vi "Create_Trajectory_Config_Parse_V1_V2_V3.vi"(8 "error in (no error)":errorcluster, 10 "Units Selector":T4, 11 "XML Elements":string) -> (0 "error out":errorcluster, 3 "TrajCreateConfig":T1 {"WayPoints"."WEIGHT" format="%13.3f"; "WayPoints"."ANGLE" format="%13.3f"; "WayPoints"."Y" format="%13.3f"; "WayPoints"."X" format="%13.3f"; "TRAJECTORY_CONFIG"."End Velocity" format="%20.4f"; "TRAJECTORY_CONFIG"."StartVelocity" format="%20.4f"; "TRAJECTORY_CONFIG"."Max Acceleration" format="%20.4f"; "TRAJECTORY_CONFIG"."MaxVelocity" format="%20.4f"})   [LabVIEW 2019]
uses:
  CreateTrajectoryENUM/TrajCreateUnitsENUM.ctl
  CreateTrajectoryTypeDef/TrajCreateConfig__V_Internal.ctl
  <vilib>/Rock Robotics/WPI/ThirdParty/JAS_Junk/TrajLib/TypeDef/DISPLAY_WEIGHTED_WAYPOINT.ctl
  <vilib>/Rock Robotics/WPI/ThirdParty/JAS_Junk/TrajLib/TypeDef/TRAJ_CONFIG.ctl
  CreateTrajectoryTypeDef/TrajCreateConfig_V5.ctl
  CreateTrajectoryTypeDef/TrajCreateTrajConfig_V4.ctl
  <vilib>/Rock Robotics/WPI/ThirdParty/JAS_Junk/TrajLib/TypeDef/TRAJ_CONSTRAINT_DIIF_DRIVE_KINEMATICS.ctl
  <vilib>/Rock Robotics/WPI/ThirdParty/JAS_Junk/TrajLib/TypeDef/DIFF_DRIVE_KINEMATICS.ctl
  <vilib>/Rock Robotics/WPI/ThirdParty/JAS_Junk/TrajLib/TypeDef/TRAJ_CONSTRAINT_CENTRIPETAL_ACCEL.ctl
  <vilib>/Rock Robotics/WPI/ThirdParty/JAS_Junk/TrajLib/TypeDef/TRAJ_CONSTRAINT_SWERVE_DRIVE_KINEMATICS.ctl
  <vilib>/Rock Robotics/WPI/ThirdParty/JAS_Junk/TrajLib/TypeDef/SWERVE_DRIVE_KINEMATICS.ctl
  <vilib>/Analysis/Matrix/Datatypes/RealMatrix.ctl
  <vilib>/Rock Robotics/WPI/ThirdParty/JAS_Junk/TrajLib/TypeDef/TRANSLATION2D.ctl
  <vilib>/Rock Robotics/WPI/ThirdParty/JAS_Junk/TrajLib/TypeDef/SWERVE_DRIVE_MODULE_STATE.ctl
  <vilib>/Rock Robotics/WPI/ThirdParty/JAS_Junk/TrajLib/TypeDef/ROTATION2D.ctl
  <vilib>/Rock Robotics/WPI/ThirdParty/JAS_Junk/TrajLib/TypeDef/TRAJ_CONSTRAINT_DIIF_DRIVE_VOLTAGE.ctl
  <vilib>/Rock Robotics/WPI/ThirdParty/JAS_Junk/TrajLib/TypeDef/SIMPLE_MOTOR_FF.ctl
  <vilib>/Rock Robotics/WPI/ThirdParty/JAS_Junk/TrajLib/TypeDef/TRAJ_CONSTRAINT_MECA_DRIVE_KINEMATICS.ctl
  <vilib>/Rock Robotics/WPI/ThirdParty/JAS_Junk/TrajLib/TypeDef/MECA_DRIVE_KINEMATICS.ctl
  CreateTrajectoryTypeDef/TrajCreateConfig_V4.ctl
  CreateTrajectoryTypeDef/TrajCreateConfig_V3.ctl
  CreateTrajectoryTypeDef/TrajCreateConfig_V2.ctl
  <vilib>/Rock Robotics/WPI/ThirdParty/JAS_Junk/TrajLib/TypeDef/DISPLAY_WAYPOINT.ctl
  CreateTrajectoryTypeDef/TrajCreateConfig_V1.ctl
  <vilib>/Rock Robotics/WPI/ThirdParty/JAS_Junk/TrajLib/Trajectory_Library.lvlib
  <vilib>/Analysis/Matrix/NI_Matrix.lvlib
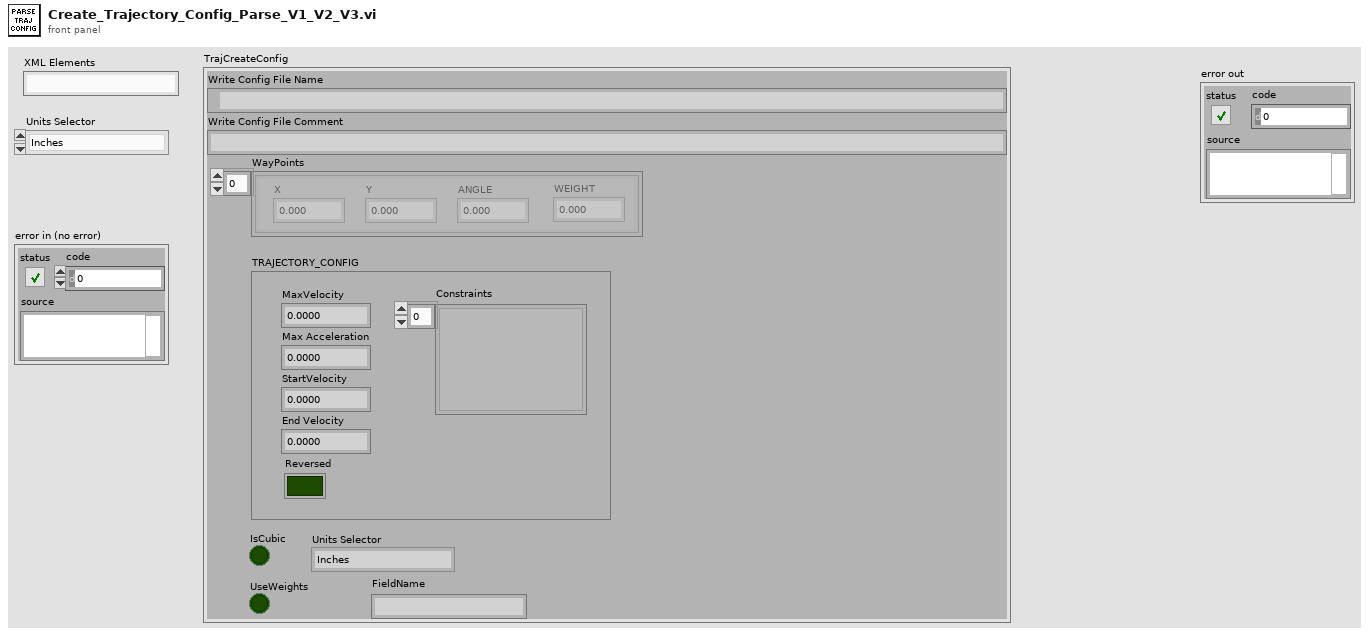
[diagram p1: front panel]
types:
  T1 = typedef "TrajCreateConfig__V_Internal.ctl" = cluster{"Write Config File Name":path, "Write Config File Comment":string, "WayPoints":T2[], "TRAJECTORY_CONFIG":T3, "IsCubic":bool, "Units Selector":T4, "UseWeights":bool, "FieldName":string}
  T2 = typedef "Trajectory_Library.lvlib/DISPLAY_WEIGHTED_WAYPOINT.ctl" = cluster{"X":dbl, "Y":dbl, "ANGLE":dbl, "WEIGHT":dbl}
  T3 = typedef "Trajectory_Library.lvlib/TRAJ_CONFIG.ctl" = cluster{"MaxVelocity":dbl, "Max Acceleration":dbl, "StartVelocity":dbl, "End Velocity":dbl, "Reversed":bool, "Constraints":variant[]}
  T4 = typedef "TrajCreateUnitsENUM.ctl" = enum16{"Inches", "Feet", "Centimeters", "Meters"}
  T5 = typedef "TrajCreateConfig_V5.ctl" = cluster{"Write Config File Name":path, "Write Config File Comment":string, "WayPoints":T2[], "TRAJECTORY_CONFIG_V4":T6, "IsCubic":bool, "Units Selector":T4, "UseWeights":bool, "FieldName":string, "Rect Region Exists":bool, "RectRegionBotLeft":T13, "RectRegionTopRight":T13, "Rect Region Max Speed":dbl}
  T6 = typedef "TrajCreateTrajConfig_V4.ctl" = cluster{"MaxVelocity":dbl, "Max Acceleration":dbl, "StartVelocity":dbl, "End Velocity":dbl, "Reversed":bool, "DiffDrKineConstntDefined":bool, "CentAcellConstntDefined":bool, "DiffDrVoltConstntDefined":bool, "DIFF_DRIVE_KINE_CONSTRAINT":T7, "CENTRIPETAL_ACCEL_CONSTRAINT":T9, "SwerveDrKineConstntDefined":bool, "SWERVE_DRIVE_KINE_CONSTRAINT":T10, "DIFF_DRIVE_VOLTAGE_CONSTRAINT":T16, "MECANUM_DRIVE_KINE_CONSTRAINT":T18, "MecanumDrKineConstntDefined":bool}
  T7 = typedef "Trajectory_Library.lvlib/TRAJ_CONSTRAINT_DIIF_DRIVE_KINEMATICS.ctl" = cluster{"Max Speed (M/S)":dbl, "DIFF_DRIVE_KINEMATICS":T8, "Max Accel (M/S2)":dbl}
  T8 = typedef "Trajectory_Library.lvlib/DIFF_DRIVE_KINEMATICS.ctl" = cluster{"TrackWidth_Meters":dbl}
  T9 = typedef "Trajectory_Library.lvlib/TRAJ_CONSTRAINT_CENTRIPETAL_ACCEL.ctl" = cluster{"Max Cent Accel":dbl}
  T10 = typedef "Trajectory_Library.lvlib/TRAJ_CONSTRAINT_SWERVE_DRIVE_KINEMATICS.ctl" = cluster{"Max Speed (M/S)":dbl, "SwerveKinematics":T11}
  T11 = typedef "Trajectory_Library.lvlib/SWERVE_DRIVE_KINEMATICS.ctl" = cluster{"NumModules":i32, "InverseKinematics":T12, "ForwardKinematics":T12, "Modules":T13[], "PrevCoR":T13, "SavedModuleStates":T14[]}
  T12 = typedef "NI_Matrix.lvlib/RealMatrix.ctl" = dbl[][]
  T13 = typedef "Trajectory_Library.lvlib/TRANSLATION2D.ctl" = cluster{"X":dbl, "Y":dbl}
  T14 = typedef "Trajectory_Library.lvlib/SWERVE_DRIVE_MODULE_STATE.ctl" = cluster{"Speed":dbl, "Angle":T15}
  T15 = typedef "Trajectory_Library.lvlib/ROTATION2D.ctl" = cluster{"VALUE":dbl, "COS":dbl, "SIN":dbl}
  T16 = typedef "Trajectory_Library.lvlib/TRAJ_CONSTRAINT_DIIF_DRIVE_VOLTAGE.ctl" = cluster{"Max Voltage":dbl, "DIFF_DRIVE_KINEMATICS":T8, "SIMPLE_MOTOR_FF":T17}
  T17 = typedef "Trajectory_Library.lvlib/SIMPLE_MOTOR_FF.ctl" = cluster{"Ks":dbl, "Kv":dbl, "Ka":dbl, "KnInv":dbl}
  T18 = typedef "Trajectory_Library.lvlib/TRAJ_CONSTRAINT_MECA_DRIVE_KINEMATICS.ctl" = cluster{"Max Speed (M/S)":dbl, "MECA_DRIVE_KINEMATICS":T19}
  T19 = typedef "Trajectory_Library.lvlib/MECA_DRIVE_KINEMATICS.ctl" = cluster{"FrontLeft":T13, "FrontRight":T13, "RearLeft":T13, "RearRight":T13, "InverseKinematics":T12, "ForwardKinematics":T12, "PrevCoR":T13}
  T20 = typedef "TrajCreateConfig_V4.ctl" = cluster{"Write Config File Name":path, "Write Config File Comment":string, "WayPoints":T2[], "TRAJECTORY_CONFIG_V4":T6, "IsCubic":bool, "Units Selector":T4, "UseWeights":bool, "FieldName":string}
  T21 = typedef "TrajCreateConfig_V3.ctl" = cluster{"Write Config File Name":path, "Write Config File Comment":string, "WayPoints":T2[], "TRAJECTORY_CONFIG":cluster{"MaxVelocity":dbl, "Max Acceleration":dbl, "StartVelocity":dbl, "End Velocity":dbl, "Reversed":bool, "DiffDrKineConstntDefined":bool, "CentAcellConstntDefined":bool, "DiffDrVoltConstntDefined":bool, "DIFF_DRIVE_KINE_CONSTRAINT":cluster{"Max Speed (M/S)":dbl, "DIFF_DRIVE_KINEMATICS":T8}, "CENTRIPETAL_ACCEL_CONSTRAINT":T9, "SwerveDrKineConstntDefined":bool, "SWERVE_DRIVE_KINE_CONSTRAINT":T10, "DIFF_DRIVE_VOLTAGE_CONSTRAINT":T16, "MECANUM_DRIVE_KINE_CONSTRAINT":T18, "MecanumDrKineConstntDefined":bool}, "IsCubic":bool, "Units Selector":T4, "UseWeights":bool}
  T22 = typedef "TrajCreateConfig_V2.ctl" = cluster{"Write Config File Name":path, "Write Config File Comment":string, "WayPoints":T23[], "TRAJECTORY_CONFIG":cluster{"MaxVelocity":dbl, "Max Acceleration":dbl, "StartVelocity":dbl, "End Velocity":dbl, "Reversed":bool, "DiffDrKineConstntDefined":bool, "CentAcellConstntDefined":bool, "DiffDrVoltConstntDefined":bool, "DIFF_DRIVE_KINE_CONSTRAINT":cluster{"Max Speed (M/S)":dbl, "DIFF_DRIVE_KINEMATICS":T8}, "CENTRIPETAL_ACCEL_CONSTRAINT":T9, "SwerveDrKineConstntDefined":bool, "SWERVE_DRIVE_KINE_CONSTRAINT":T10, "DIFF_DRIVE_VOLTAGE_CONSTRAINT":T16, "MECANUM_DRIVE_KINE_CONSTRAINT":T18, "MecanumDrKineConstntDefined":bool}, "IsCubic":bool, "Units Selector":T4}
  T23 = typedef "Trajectory_Library.lvlib/DISPLAY_WAYPOINT.ctl" = cluster{"X":dbl, "Y":dbl, "ANGLE":dbl}
  T24 = typedef "TrajCreateConfig_V1.ctl" = cluster{"Write Config File Name":path, "Write Config File Comment":string, "WayPoints":T23[], "TRAJECTORY_CONFIG":cluster{"MaxVelocity":dbl, "Max Acceleration":dbl, "StartVelocity":dbl, "End Velocity":dbl, "Reversed":bool, "DiffDrKineConstntDefined":bool, "CentAcellConstntDefined":bool, "DiffDrVoltConstntDefined":bool, "DIFF_DRIVE_KINE_CONSTRAINT":cluster{"Max Speed (M/S)":dbl, "DIFF_DRIVE_KINEMATICS":T8}, "CENTRIPETAL_ACCEL_CONSTRAINT":T9, "SwerveDrKineConstntDefined":bool, "SWERVE_DRIVE_KINE_CONSTRAINT":T10, "DIFF_DRIVE_VOLTAGE_CONSTRAINT":T16, "MECANUM_DRIVE_KINE_CONSTRAINT":T18, "MecanumDrKineConstntDefined":bool}, "IsCubic":bool}
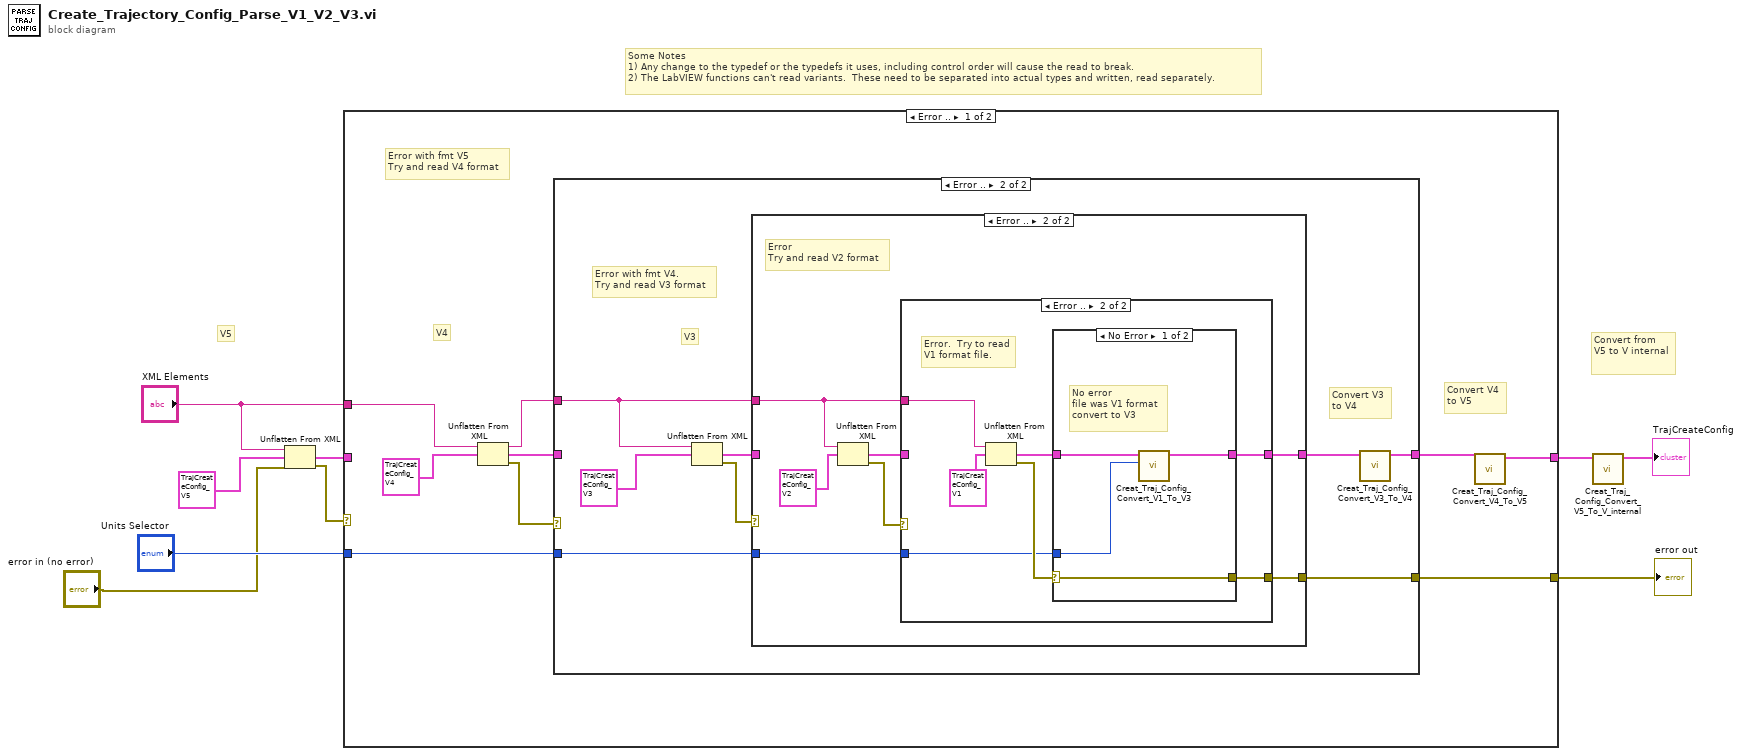
[diagram p0: block diagram]
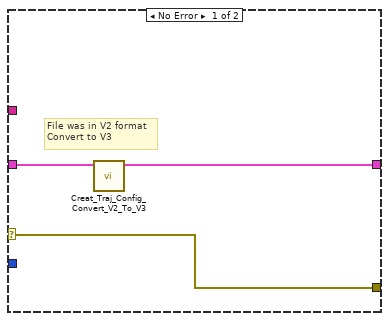
[diagram p4: hidden frame]
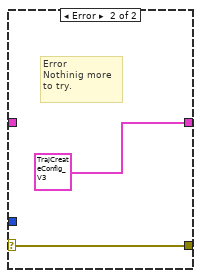
[diagram p5: hidden frame]
diagram:
  # "V5"
  # "Convert from\nV5 to V internal"
  # "Some Notes\n1) Any change to the typedef or the typedefs it uses, including control order will cause the read to break.\n2) The LabVIEW functions can't read variants.  These need to be separated into actual types and written, read separately."
  n1 = Unflatten From XML(xml string="XML Elements", type=T5 {"Write Config File Name"=path "", "Write Config File Comment"="", "WayPoints"=[], "TRAJECTORY_CONFIG_V4"={"MaxVelocity"=0.0, "Max Acceleration"=0.0, "StartVelocity"=0.0, "End Velocity"=0.0, "Reversed"=FALSE, "DiffDrKineConstntDefined"=FALSE, "CentAcellConstntDefined"=FALSE, "DiffDrVoltConstntDefined"=FALSE, "DIFF_DRIVE_KINE_CONSTRAINT"={"Max Speed (M/S)"=0.0, "DIFF_DRIVE_KINEMATICS"={"TrackWidth_Meters"=0.0}, "Max Accel (M/S2)"=99999.0}, "CENTRIPETAL_ACCEL_CONSTRAINT"={"Max Cent Accel"=0.0}, "SwerveDrKineConstntDefined"=FALSE, "SWERVE_DRIVE_KINE_CONSTRAINT"={"Max Speed (M/S)"=0.0, "SwerveKinematics"={"NumModules"=0, "InverseKinematics"=[], "ForwardKinematics"=[], "Modules"=[], "PrevCoR"={"X"=0.0, "Y"=0.0}, "SavedModuleStates"=[]}}, "DIFF_DRIVE_VOLTAGE_CONSTRAINT"={"Max Voltage"=0.0, "DIFF_DRIVE_KINEMATICS"={"TrackWidth_Meters"=0.0}, "SIMPLE_MOTOR_FF"={"Ks"=0.0, "Kv"=0.0, "Ka"=0.0, "KnInv"=0.0}}, "MECANUM_DRIVE_KINE_CONSTRAINT"={"Max Speed (M/S)"=0.0, "MECA_DRIVE_KINEMATICS"={"FrontLeft"={"X"=0.0, "Y"=0.0}, "FrontRight"={"X"=0.0, "Y"=0.0}, "RearLeft"={"X"=0.0, "Y"=0.0}, "RearRight"={"X"=0.0, "Y"=0.0}, "InverseKinematics"=[[0.0, 1.0, -1.0, 0.0], [0.0, 1.0, 1.0, 0.0], [0.0, 1.0, 1.0, 0.0], [0.0, 1.0, -1.0, 0.0]], "ForwardKinematics"=[[0.0, 1.0, -1.0, 0.0], [0.0, 1.0, 1.0, 0.0], [0.0, 1.0, 1.0, 0.0], [0.0, 1.0, -1.0, 0.0]], "PrevCoR"={"X"=0.0, "Y"=0.0}}}, "MecanumDrKineConstntDefined"=FALSE}, "IsCubic"=FALSE, "Units Selector"=enum."Inches", "UseWeights"=FALSE, "FieldName"="", "Rect Region Exists"=FALSE, "RectRegionBotLeft"={"X"=0.0, "Y"=0.0}, "RectRegionTopRight"={"X"=0.0, "Y"=0.0}, "Rect Region Max Speed"=0.0} ("TrajCreateConfigV5"), error in (no error)="error in (no error)") -> (value=w2:T5, error out=w6:errorcluster)
  n2 = case shown="Error .." w6 {
    selector: w6 -> [_ w53]
    tunnel: "Units Selector" -> [w17 _]
    tunnel: [w16 w53] -> w8
    tunnel: "XML Elements" -> [w13 _]
    tunnel: w2 -> [_ w54]
    tunnel: [w10 w54] -> w1
    frame Error {
      # "V4"
      # "Convert V4\nto V5"
      # "Error with fmt V5\nTry and read V4 format"
      n3 = Unflatten From XML(xml string=w13, type=T20 {"Write Config File Name"=path "", "Write Config File Comment"="", "WayPoints"=[], "TRAJECTORY_CONFIG_V4"={"MaxVelocity"=0.0, "Max Acceleration"=0.0, "StartVelocity"=0.0, "End Velocity"=0.0, "Reversed"=FALSE, "DiffDrKineConstntDefined"=FALSE, "CentAcellConstntDefined"=FALSE, "DiffDrVoltConstntDefined"=FALSE, "DIFF_DRIVE_KINE_CONSTRAINT"={"Max Speed (M/S)"=0.0, "DIFF_DRIVE_KINEMATICS"={"TrackWidth_Meters"=0.0}, "Max Accel (M/S2)"=99999.0}, "CENTRIPETAL_ACCEL_CONSTRAINT"={"Max Cent Accel"=0.0}, "SwerveDrKineConstntDefined"=FALSE, "SWERVE_DRIVE_KINE_CONSTRAINT"={"Max Speed (M/S)"=0.0, "SwerveKinematics"={"NumModules"=0, "InverseKinematics"=[], "ForwardKinematics"=[], "Modules"=[], "PrevCoR"={"X"=0.0, "Y"=0.0}, "SavedModuleStates"=[]}}, "DIFF_DRIVE_VOLTAGE_CONSTRAINT"={"Max Voltage"=0.0, "DIFF_DRIVE_KINEMATICS"={"TrackWidth_Meters"=0.0}, "SIMPLE_MOTOR_FF"={"Ks"=0.0, "Kv"=0.0, "Ka"=0.0, "KnInv"=0.0}}, "MECANUM_DRIVE_KINE_CONSTRAINT"={"Max Speed (M/S)"=0.0, "MECA_DRIVE_KINEMATICS"={"FrontLeft"={"X"=0.0, "Y"=0.0}, "FrontRight"={"X"=0.0, "Y"=0.0}, "RearLeft"={"X"=0.0, "Y"=0.0}, "RearRight"={"X"=0.0, "Y"=0.0}, "InverseKinematics"=[[0.0, 1.0, -1.0, 0.0], [0.0, 1.0, 1.0, 0.0], [0.0, 1.0, 1.0, 0.0], [0.0, 1.0, -1.0, 0.0]], "ForwardKinematics"=[[0.0, 1.0, -1.0, 0.0], [0.0, 1.0, 1.0, 0.0], [0.0, 1.0, 1.0, 0.0], [0.0, 1.0, -1.0, 0.0]], "PrevCoR"={"X"=0.0, "Y"=0.0}}}, "MecanumDrKineConstntDefined"=FALSE}, "IsCubic"=FALSE, "Units Selector"=enum."Inches", "UseWeights"=FALSE, "FieldName"=""} ("TrajCreateConfig")) -> (value=w12:T20, error out=w14:errorcluster)  [unwired: 1 in]
      n4 = case shown="Error .." w14 {
        selector: w14 -> [w18 _]
        tunnel: w17 -> [_ w27]
        tunnel: [w18 w26] -> w16
        tunnel: w13 -> [_ w22]
        tunnel: [w19 w20] -> w11
        tunnel: w12 -> [w19 _]
        frame No Error {
          # "No Error -- File was in V4 Format"
        }
        frame Error {
          # "Convert V3\nto V4"
          # "Error with fmt V4.\nTry and read V3 format"
          # "V3"
          n5 = Unflatten From XML(xml string=w22, type=T21 {"Write Config File Name"=path "", "Write Config File Comment"="", "WayPoints"=[], "TRAJECTORY_CONFIG"={"MaxVelocity"=0.0, "Max Acceleration"=0.0, "StartVelocity"=0.0, "End Velocity"=0.0, "Reversed"=FALSE, "DiffDrKineConstntDefined"=FALSE, "CentAcellConstntDefined"=FALSE, "DiffDrVoltConstntDefined"=FALSE, "DIFF_DRIVE_KINE_CONSTRAINT"={"Max Speed (M/S)"=0.0, "DIFF_DRIVE_KINEMATICS"={"TrackWidth_Meters"=0.0}}, "CENTRIPETAL_ACCEL_CONSTRAINT"={"Max Cent Accel"=0.0}, "SwerveDrKineConstntDefined"=FALSE, "SWERVE_DRIVE_KINE_CONSTRAINT"={"Max Speed (M/S)"=0.0, "SwerveKinematics"={"NumModules"=0, "InverseKinematics"=[], "ForwardKinematics"=[], "Modules"=[], "PrevCoR"={"X"=0.0, "Y"=0.0}, "SavedModuleStates"=[]}}, "DIFF_DRIVE_VOLTAGE_CONSTRAINT"={"Max Voltage"=0.0, "DIFF_DRIVE_KINEMATICS"={"TrackWidth_Meters"=0.0}, "SIMPLE_MOTOR_FF"={"Ks"=0.0, "Kv"=0.0, "Ka"=0.0, "KnInv"=0.0}}, "MECANUM_DRIVE_KINE_CONSTRAINT"={"Max Speed (M/S)"=0.0, "MECA_DRIVE_KINEMATICS"={"FrontLeft"={"X"=0.0, "Y"=0.0}, "FrontRight"={"X"=0.0, "Y"=0.0}, "RearLeft"={"X"=0.0, "Y"=0.0}, "RearRight"={"X"=0.0, "Y"=0.0}, "InverseKinematics"=[], "ForwardKinematics"=[], "PrevCoR"={"X"=0.0, "Y"=0.0}}}, "MecanumDrKineConstntDefined"=FALSE}, "IsCubic"=FALSE, "Units Selector"=enum."Inches", "UseWeights"=FALSE} ("TrajCreateConfig")) -> (value=w24:T21, error out=w23:errorcluster)  [unwired: 1 in]
          n6 = case shown="Error .." w23 {
            selector: w23 -> [w29 _]
            tunnel: [w29 w32] -> w26
            tunnel: w27 -> [_ w34]
            tunnel: w24 -> [w28 _]
            tunnel: [w28 w31] -> w21
            tunnel: w22 -> [_ w30]
            frame No Error {
              # "No Error.  File was V3\nformat."
            }
            frame Error {
              # "Error\nTry and read V2 format"
              n7 = Unflatten From XML(xml string=w30, type=T22 {"Write Config File Name"=path "", "Write Config File Comment"="", "WayPoints"=[], "TRAJECTORY_CONFIG"={"MaxVelocity"=0.0, "Max Acceleration"=0.0, "StartVelocity"=0.0, "End Velocity"=0.0, "Reversed"=FALSE, "DiffDrKineConstntDefined"=FALSE, "CentAcellConstntDefined"=FALSE, "DiffDrVoltConstntDefined"=FALSE, "DIFF_DRIVE_KINE_CONSTRAINT"={"Max Speed (M/S)"=0.0, "DIFF_DRIVE_KINEMATICS"={"TrackWidth_Meters"=0.0}}, "CENTRIPETAL_ACCEL_CONSTRAINT"={"Max Cent Accel"=0.0}, "SwerveDrKineConstntDefined"=FALSE, "SWERVE_DRIVE_KINE_CONSTRAINT"={"Max Speed (M/S)"=0.0, "SwerveKinematics"={"NumModules"=0, "InverseKinematics"=[], "ForwardKinematics"=[], "Modules"=[], "PrevCoR"={"X"=0.0, "Y"=0.0}, "SavedModuleStates"=[]}}, "DIFF_DRIVE_VOLTAGE_CONSTRAINT"={"Max Voltage"=0.0, "DIFF_DRIVE_KINEMATICS"={"TrackWidth_Meters"=0.0}, "SIMPLE_MOTOR_FF"={"Ks"=0.0, "Kv"=0.0, "Ka"=0.0, "KnInv"=0.0}}, "MECANUM_DRIVE_KINE_CONSTRAINT"={"Max Speed (M/S)"=0.0, "MECA_DRIVE_KINEMATICS"={"FrontLeft"={"X"=0.0, "Y"=0.0}, "FrontRight"={"X"=0.0, "Y"=0.0}, "RearLeft"={"X"=0.0, "Y"=0.0}, "RearRight"={"X"=0.0, "Y"=0.0}, "InverseKinematics"=[], "ForwardKinematics"=[], "PrevCoR"={"X"=0.0, "Y"=0.0}}}, "MecanumDrKineConstntDefined"=FALSE}, "IsCubic"=FALSE, "Units Selector"=enum."Inches"} ("TrajCreateConfig")) -> (value=w35:T22, error out=w33:errorcluster)  [unwired: 1 in]
              n8 = case shown="Error .." w33 {
                selector: w33 -> [w38 _]
                tunnel: w35 -> [w39 _]
                tunnel: w34 -> [_ w41]
                tunnel: [w38 w43] -> w32
                tunnel: [w37 w42] -> w31
                tunnel: w30 -> [_ w45]
                frame No Error {
                  # "File was in V2 format\nConvert to V3"
                  n9 = call "Creat_Traj_Config_Convert_V2_To_V3.vi"("TrajCreateConfig in"=w39) -> ("TrajCreateConfig out"=w37:T21)  [unwired: 10 in]
                }
                frame Error {
                  # "Error.  Try to read\nV1 format file."
                  n10 = Unflatten From XML(xml string=w45, type=T24 {"Write Config File Name"=path "", "Write Config File Comment"="", "WayPoints"=[], "TRAJECTORY_CONFIG"={"MaxVelocity"=0.0, "Max Acceleration"=0.0, "StartVelocity"=0.0, "End Velocity"=0.0, "Reversed"=FALSE, "DiffDrKineConstntDefined"=FALSE, "CentAcellConstntDefined"=FALSE, "DiffDrVoltConstntDefined"=FALSE, "DIFF_DRIVE_KINE_CONSTRAINT"={"Max Speed (M/S)"=0.0, "DIFF_DRIVE_KINEMATICS"={"TrackWidth_Meters"=0.0}}, "CENTRIPETAL_ACCEL_CONSTRAINT"={"Max Cent Accel"=0.0}, "SwerveDrKineConstntDefined"=FALSE, "SWERVE_DRIVE_KINE_CONSTRAINT"={"Max Speed (M/S)"=0.0, "SwerveKinematics"={"NumModules"=0, "InverseKinematics"=[], "ForwardKinematics"=[], "Modules"=[], "PrevCoR"={"X"=0.0, "Y"=0.0}, "SavedModuleStates"=[]}}, "DIFF_DRIVE_VOLTAGE_CONSTRAINT"={"Max Voltage"=0.0, "DIFF_DRIVE_KINEMATICS"={"TrackWidth_Meters"=0.0}, "SIMPLE_MOTOR_FF"={"Ks"=0.0, "Kv"=0.0, "Ka"=0.0, "KnInv"=0.0}}, "MECANUM_DRIVE_KINE_CONSTRAINT"={"Max Speed (M/S)"=0.0, "MECA_DRIVE_KINEMATICS"={"FrontLeft"={"X"=0.0, "Y"=0.0}, "FrontRight"={"X"=0.0, "Y"=0.0}, "RearLeft"={"X"=0.0, "Y"=0.0}, "RearRight"={"X"=0.0, "Y"=0.0}, "InverseKinematics"=[], "ForwardKinematics"=[], "PrevCoR"={"X"=0.0, "Y"=0.0}}}, "MecanumDrKineConstntDefined"=FALSE}, "IsCubic"=FALSE} ("TrajCreateConfig")) -> (value=w40:T24, error out=w44:errorcluster)  [unwired: 1 in]
                  n11 = case shown="No Error" w44 {
                    selector: w44 -> [w50 w52]
                    tunnel: [w50 w52] -> w43
                    tunnel: [w49 T21 {"Write Config File Name"=path "", "Write Config File Comment"="", "WayPoints"=[], "TRAJECTORY_CONFIG"={"MaxVelocity"=0.0, "Max Acceleration"=0.0, "StartVelocity"=0.0, "End Velocity"=0.0, "Reversed"=FALSE, "DiffDrKineConstntDefined"=FALSE, "CentAcellConstntDefined"=FALSE, "DiffDrVoltConstntDefined"=FALSE, "DIFF_DRIVE_KINE_CONSTRAINT"={"Max Speed (M/S)"=0.0, "DIFF_DRIVE_KINEMATICS"={"TrackWidth_Meters"=0.0}}, "CENTRIPETAL_ACCEL_CONSTRAINT"={"Max Cent Accel"=0.0}, "SwerveDrKineConstntDefined"=FALSE, "SWERVE_DRIVE_KINE_CONSTRAINT"={"Max Speed (M/S)"=0.0, "SwerveKinematics"={"NumModules"=0, "InverseKinematics"=[], "ForwardKinematics"=[], "Modules"=[], "PrevCoR"={"X"=0.0, "Y"=0.0}, "SavedModuleStates"=[]}}, "DIFF_DRIVE_VOLTAGE_CONSTRAINT"={"Max Voltage"=0.0, "DIFF_DRIVE_KINEMATICS"={"TrackWidth_Meters"=0.0}, "SIMPLE_MOTOR_FF"={"Ks"=0.0, "Kv"=0.0, "Ka"=0.0, "KnInv"=0.0}}, "MECANUM_DRIVE_KINE_CONSTRAINT"={"Max Speed (M/S)"=0.0, "MECA_DRIVE_KINEMATICS"={"FrontLeft"={"X"=0.0, "Y"=0.0}, "FrontRight"={"X"=0.0, "Y"=0.0}, "RearLeft"={"X"=0.0, "Y"=0.0}, "RearRight"={"X"=0.0, "Y"=0.0}, "InverseKinematics"=[], "ForwardKinematics"=[], "PrevCoR"={"X"=0.0, "Y"=0.0}}}, "MecanumDrKineConstntDefined"=FALSE}, "IsCubic"=FALSE, "Units Selector"=enum."Inches", "UseWeights"=FALSE} ("TrajCreateConfig")] -> w42
                    tunnel: w41 -> [w48 _]
                    tunnel: w40 -> [w47 _]
                    frame No Error {
                      # "No error\nfile was V1 format\nconvert to V3"
                      n12 = call "Creat_Traj_Config_Convert_V1_To_V3.vi"("Units Selector"=w48, "TrajCreateConfig in"=w47) -> ("TrajCreateConfig out"=w49:T21)  [unwired: 9 in]
                    }
                    frame Error {
                      # "Error\nNothinig more\nto try."
                    }
                  }
                }
              }
            }
          }
          n13 = call "Creat_Traj_Config_Convert_V3_To_V4.vi"("TrajCreateConfig in"=w21) -> ("TrajCreateConfig out"=w20:T20)  [unwired: 10 in]
        }
      }
      n14 = call "Creat_Traj_Config_Convert_V4_To_V5.vi"("TrajCreateConfig V4 in"=w11) -> ("TrajCreateConfig V5 out"=w10:T5)  [unwired: 10 in]
    }
    frame No Error {
    }
  }
  "error out" <- w8
  n15 = call "Creat_Traj_Config_Convert_V5_To_V_internal.vi"("TrajCreateConfig V5"=w1) -> ("TrajCreateConfig V_Internal"=→"TrajCreateConfig":T1)  [unwired: 10 in]
